vi "Hood Controller.vi"(8 "error in":errorcluster) -> ()   [LabVIEW 2019]
doc: "This VI executes continuously carrying out the current operation and responding to updates or new operations. It will often contain the timing or control code that is difficult to place directly in TeleOp. This VI generally opens all sensors and motors and isolates the rest of the robot code from knowing how the operations are carried out."
uses:
  <vilib>/Rock Robotics/WPI/Framework/Completion Status.ctl
  Hood Setpoints.ctl
  Hood Operations.ctl
  <vilib>/Rock Robotics/WPI/ThirdParty/REV Robotics/SPARK MAX/Typedef/Spark MAX Smart Motion Parameters.ctl
  <vilib>/Rock Robotics/WPI/ThirdParty/REV Robotics/SPARK MAX/Typedef/Spark MAX Control Type.ctl
  <vilib>/Rock Robotics/WPI/MotorControl/WPI_MotorControlDeviceRef.ctl
  <vilib>/Rock Robotics/WPI/MotorControl/WPI_MotorControlType.ctl
  <vilib>/Rock Robotics/SystemInterfaces/DIO/FPGA_DIOPWMChannel.ctl
  <vilib>/Rock Robotics/WPI/PWM/WPI_PWMDeadband.ctl
  <vilib>/Rock Robotics/SystemInterfaces/DIO/FPGA_DIOChannel.ctl
  <vilib>/Rock Robotics/WPI/ThirdParty/REV Robotics/SPARK MAX/Typedef/Spark MAX Motor Type.ctl
  <vilib>/Rock Robotics/WPI/ThirdParty/REV Robotics/SPARK MAX/Typedef/Spark MAX Limit Direction.ctl
panel:
  in  "Control Mode":T1=enum."Smart Motion"
  in  "Velocity PID Constants":T2={"P Gain"=2e-05, "I Gain"=0.0, "D Gain"=0.0, "F Gain"=0.0001, "I Zone"=0.0, "Min Output"=-1.0, "Max Output"=1.0} {"Max Output" min=-1.0 max=1.0 step=0.01; "Min Output" min=-1.0 max=1.0 step=0.01; "I Zone" step=0.01; "F Gain" step=0.01; "D Gain" step=0.01; "I Gain" step=0.01; "P Gain" min=0.0 step=0.01}
  in  "Smart Motion Parameters":T3={"Max Velocity"=5600.0, "Max Acceleration"=10000.0, "Minimum Velocity Output"=0.0, "Allowed Closed Loop Error"=0.001}
  in  "D Filter":dbl(slide) scale=0.0..1.0
  out "Waveform Chart":T4(graph)={"Sensor Position"=0.28571414947509766, "Sensor Velocity"=0.0, "Setpoint"=0.0}
  in  "Interactive Values":T5={"Operation"=enum."Hood Setpoint", "Setpoint"=20.0, "Duration"=0.0}
  out "Current\nCmd":string="Started at  20:35:17.047\nDefault: Reserve,  S 0.0, D 0.000000"
  in  "Buttons":cluster{"Execute Cmd":bool, "Abort Cmd":bool}
  out "Command Timing":cluster{"Start Time (ms)":u32, "Iterations":i32}={"Start Time (ms)"=6528456, "Iterations"=0}
  out "Status":T7
  # "Interactive Command: You may fill in the settings for a command\nand schedule it with the Execute button. You can observe and abort\nany command while fine tuning the code for the controller."
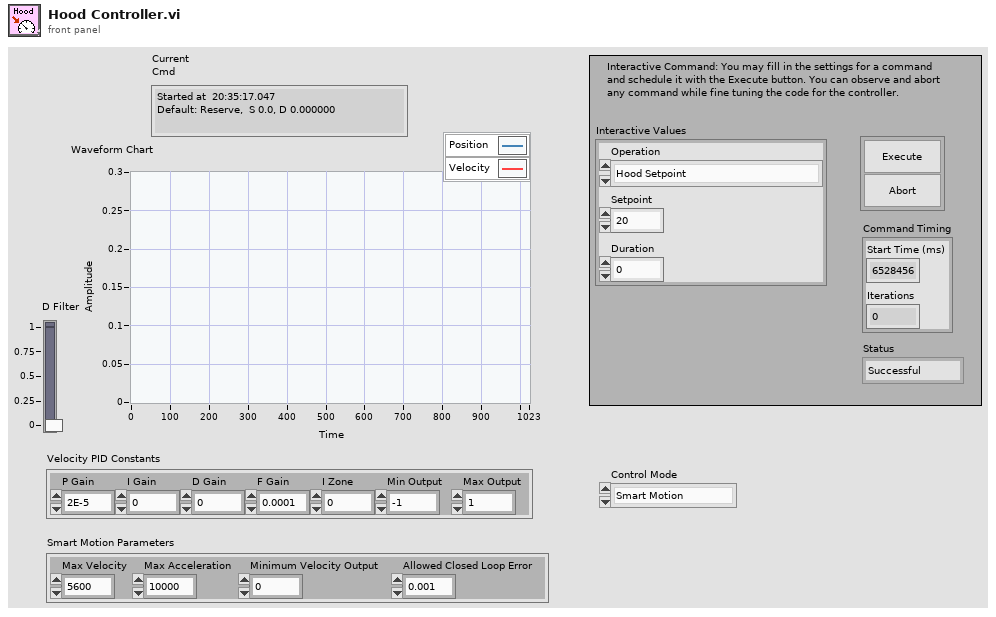
[diagram p1: front panel]
types:
  T1 = typedef "Spark MAX Control Type.ctl" = enum16{"Percent VBus", "Voltage", "Velocity", "Position", "Smart Motion", "Current", "Smart Velocity"}
  T2 = cluster{"P Gain":dbl, "I Gain":dbl, "D Gain":dbl, "F Gain":dbl, "I Zone":dbl, "Min Output":dbl, "Max Output":dbl}
  T3 = typedef "Spark MAX Smart Motion Parameters.ctl" = cluster{"Max Velocity":dbl, "Max Acceleration":dbl, "Minimum Velocity Output":dbl, "Allowed Closed Loop Error":dbl}
  T4 = cluster{"Sensor Position":dbl, "Sensor Velocity":dbl, "Setpoint":dbl}
  T5 = typedef "Hood Setpoints.ctl" = cluster{"Operation":T6, "Setpoint":dbl, "Duration":dbl}
  T6 = typedef "Hood Operations.ctl" = enum16{"Reserve", "Read Current", "Immediate", "Hood Down", "Hood Score", "Hood Setpoint"}
  T7 = typedef "Completion Status.ctl" = enum16{"Successful", "Aborted", "Incomplete"}
  T8 = typedef "Spark MAX Limit Direction.ctl" = enum16{"Forward Limit", "Reverse Limit"}
  T9 = typedef "Spark MAX Motor Type.ctl" = enum16{"Brushed", "Brushless"}
  T10 = typedef "WPI_MotorControlDeviceRef.ctl" = cluster{"DeviceStatus":errorcluster, "Type":T11, "PWM":cluster{"PWM Channel":T12, "DeadBand":T13}, "CAN":cluster{"Device Number":u8, "SetOutput VI Ref":variant, "GetOutput VI Ref":variant, "Enable VI Ref":variant, "Disable VI Ref":variant, "Data":variant}, "Invert":bool, "DIO PWM":cluster{"PWM \"Enable\" Channel":T12, "DIOChannel":T14, "PWM Rate":dbl}}
  T11 = typedef "WPI_MotorControlType.ctl" = enum16{"PWM", "CAN", "DIO PWM"}
  T12 = typedef "FPGA_DIOPWMChannel.ctl" = enum8{"PWM 0", "PWM 1", "PWM 2", "PWM 3", "PWM 4", "PWM 5", "PWM 6", "PWM 7", "PWM 8", "PWM 9", "PWM MXP 0", "PWM MXP 1", "PWM MXP 2", "PWM MXP 3", "PWM MXP 4", "PWM MXP 5", "PWM MXP 6", "PWM MXP 7", "PWM MXP 8", "PWM MXP 9", "Invalid"}
  T13 = typedef "WPI_PWMDeadband.ctl" = cluster{"Name":string, "maxPositivePwm":i32, "minPositivePwm":i32, "centerPwm":i32, "maxNegativePwm":i32, "minNegativePwm":i32, "angularRange":u16}
  T14 = typedef "FPGA_DIOChannel.ctl" = enum8{"DIO 0", "DIO 1", "DIO 2", "DIO 3", "DIO 4", "DIO 5", "DIO 6", "DIO 7", "DIO 8", "DIO 9", "DIO MXP 0", "DIO MXP 1", "DIO MXP 2", "DIO MXP 3", "DIO MXP 4", "DIO MXP 5", "DIO MXP 6", "DIO MXP 7", "DIO MXP 8", "DIO MXP 9", "DIO MXP 10", "DIO MXP 11", "DIO MXP 12", "DIO MXP 13", "DIO MXP 14", "DIO MXP 15", "SPI Port CS1", "SPI Port CS2", "SPI Port CS3", "SPI Port MISO", "SPI Port MOSI", "Invalid"}
  T15 = typedef "Command Status Info.ctl" = cluster{"Name":string, "Status":T7, "notifier out":T16}
  T16 = typedef "Completion Notifier.ctl" = refnum<notifier>
  T17 = cluster{"Current Command":T5, "Command Timing":cluster{"Start Time (ms)":u32, "Iterations":i32}, "Command Arguments":cluster{"Command Info":T15, "Description":string, "Default Command":T5, "queue out":refnum<queue>, "Subsystem Name":string}}
  T18 = cluster{"P Gain":bool, "I Gain":bool, "D Gain":bool, "F Gain":bool, "I Zone":bool, "Min Output":bool, "Max Output":bool}
  T19 = cluster{"Max Velocity":bool, "Max Acceleration":bool, "Minimum Velocity Output":bool, "Allowed Closed Loop Error":bool}
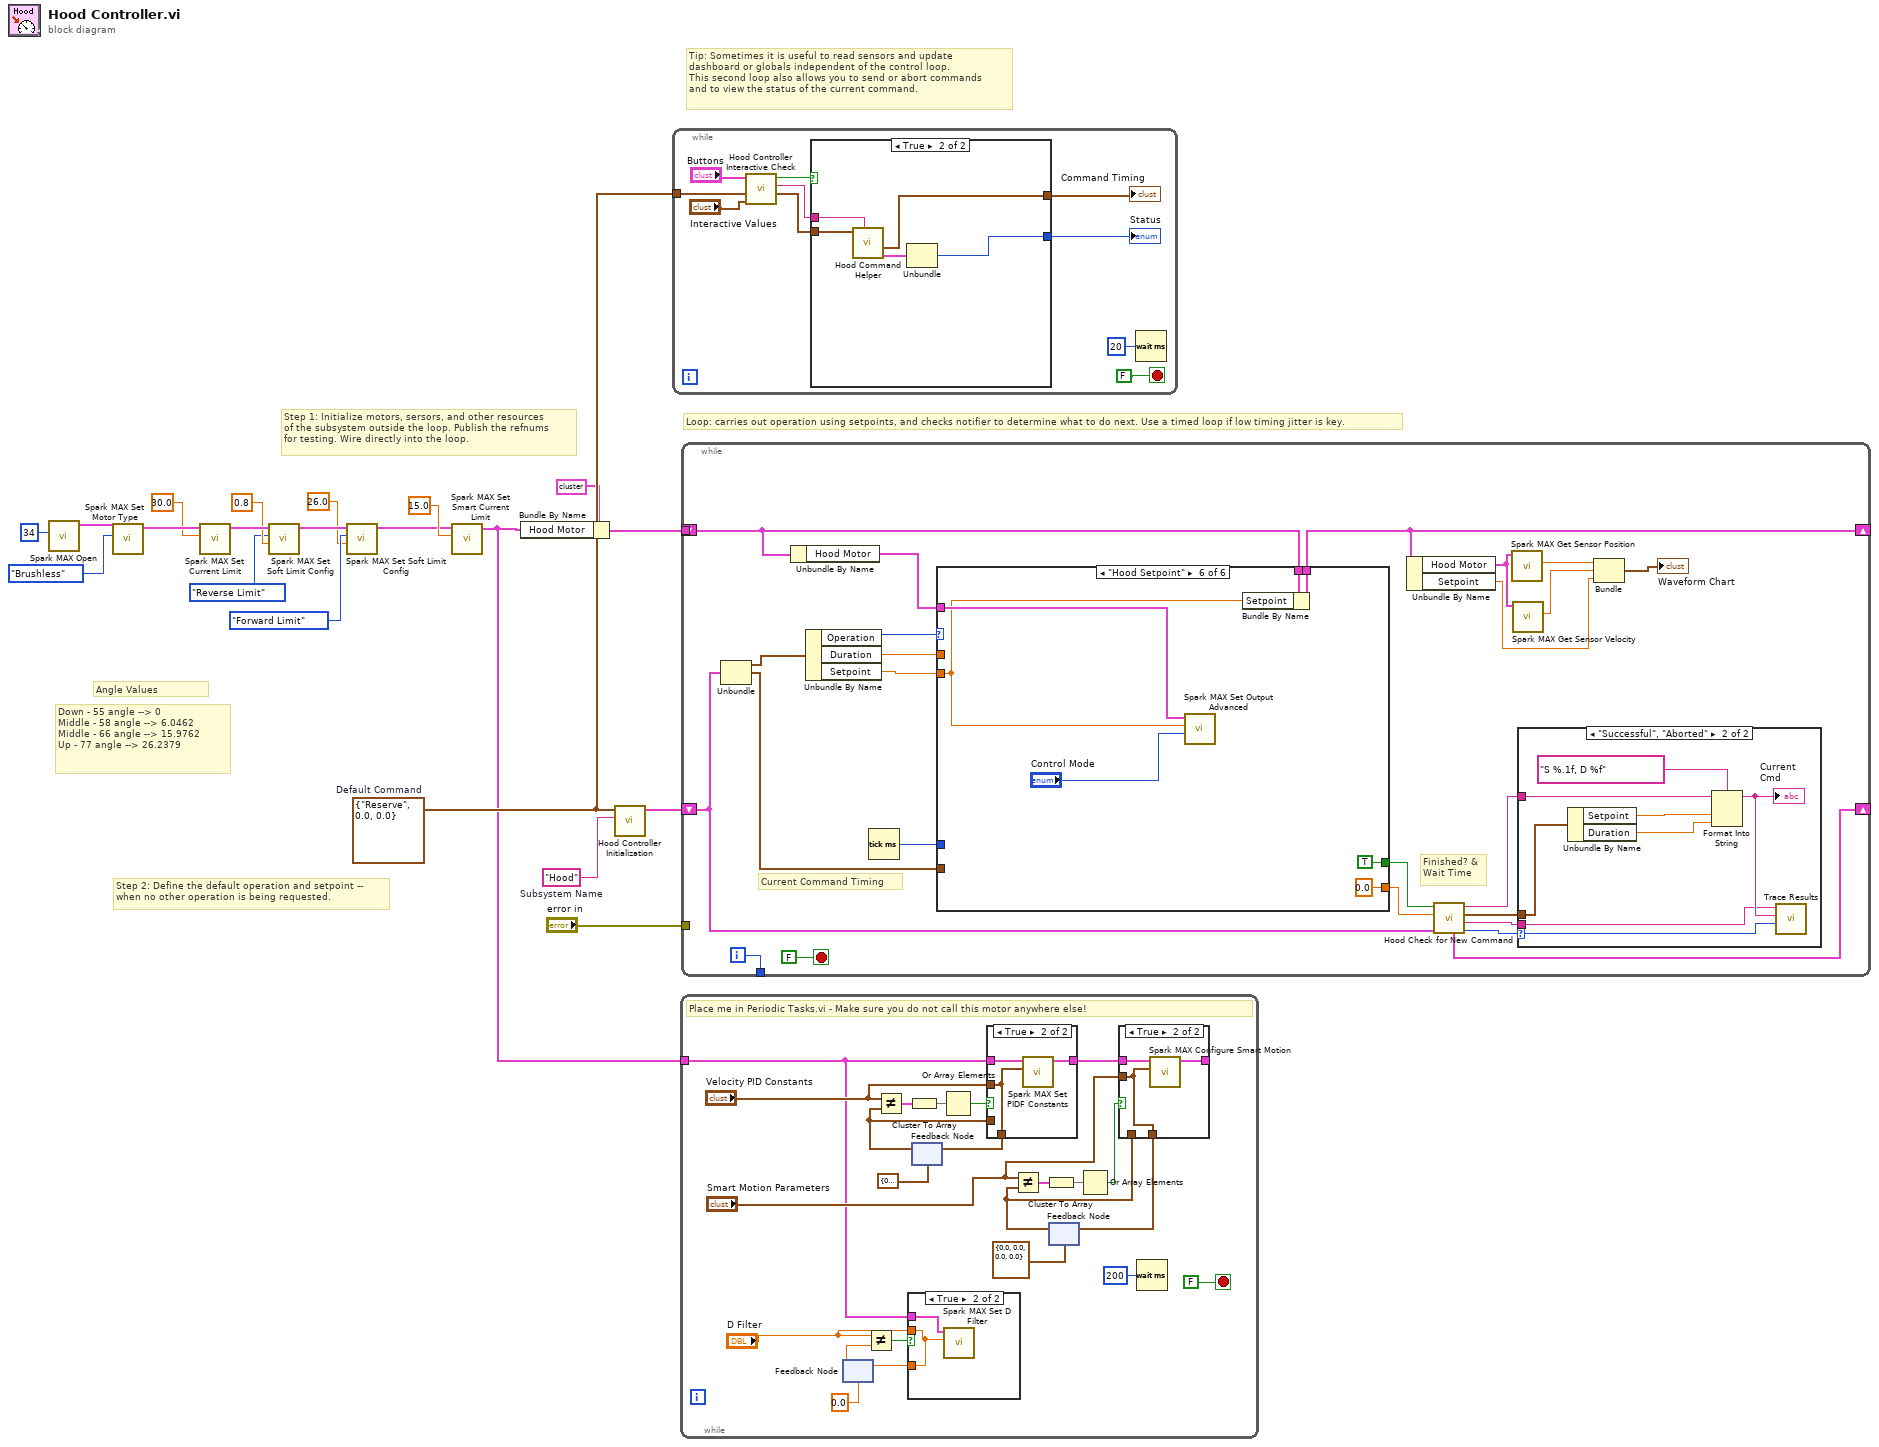
[diagram p0: block diagram]
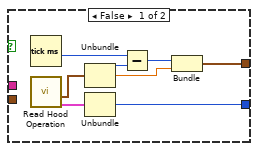
[diagram p5: hidden frame]
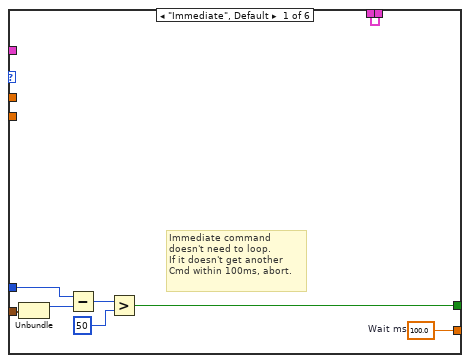
[diagram p7: hidden frame]
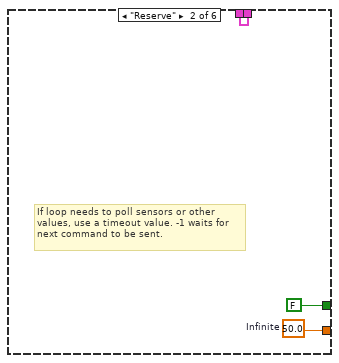
[diagram p8: hidden frame]
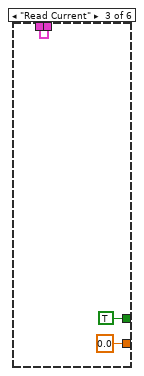
[diagram p9: hidden frame]
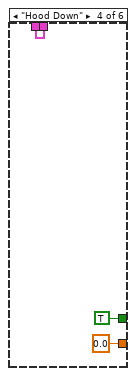
[diagram p10: hidden frame]
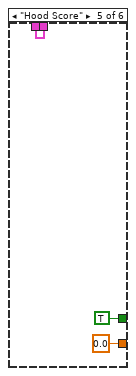
[diagram p11: hidden frame]
diagram:
  w17 = T5 {"Operation"=enum."Reserve", "Setpoint"=0.0, "Duration"=0.0}  # Default Command
  w18 = "Hood"  # Subsystem Name
  # "Angle Values"
  # "Down - 55 angle --> 0\nMiddle - 58 angle --> 6.0462\nMiddle - 66 angle --> 15.9762\nUp - 77 angle --> 26.2379"
  # "Tip: Sometimes it is useful to read sensors and update\ndashboard or globals independent of the control loop.\nThis second loop also allows you to send or abort commands\nand to view the status of the current command."
  # "Step 2: Define the default operation and setpoint --\nwhen no other operation is being requested."
  # "Step 1: Initialize motors, sersors, and other resources\nof the subsystem outside the loop. Publish the refnums\nfor testing. Wire directly into the loop."
  # "Loop: carries out operation using setpoints, and checks notifier to determine what to do next. Use a timed loop if low timing jitter is key."
  n1 = call <vilib>:"Spark MAX Open.vi"("Device Number"=u8 34) -> ("MotorControlDeviceRef"=w11:T10)  [unwired: 9 in, 1 out]
  n2 = call <vilib>:"Spark MAX Set Motor Type.vi"("Motor Type"=Spark_MAX_Motor_Type."Brushless", "MotorControlDevRef"=w11) -> ("MotorControlDeviceRef"=w15:T10)  [unwired: 8 in, 1 out]
  n3 = call <vilib>:"Spark MAX Set Current Limit.vi"("Current Limit A (100)"=sgl 30.0, "MotorControlDeviceRef in"=w15) -> ("MotorControlDeviceRef out"=w8:T10)  [unwired: 8 in, 1 out]
  n4 = call <vilib>:"Spark MAX Set Soft Limit Config.vi"("Soft Limit (0)"=0.8, "Soft Limit Switch"=Spark_MAX_Limit_Direction."Reverse Limit", "MotorControlDeviceRef in"=w8) -> ("MotorControlDeviceRef out"=w7:T10)  [unwired: 7 in, 1 out]
  n5 = call <vilib>:"Spark MAX Set Soft Limit Config.vi"("Soft Limit (0)"=26.0, "Soft Limit Switch"=Spark_MAX_Limit_Direction."Forward Limit", "MotorControlDeviceRef in"=w7) -> ("MotorControlDeviceRef out"=w4:T10)  [unwired: 7 in, 1 out]
  n6 = call <vilib>:"Spark MAX Set Smart Current Limit.vi"("Primay Current Limit (80A)"=15.0, "MotorControlDeviceRef in"=w4) -> ("MotorControlDeviceRef out"=w1:T10)  [unwired: 8 in, 1 out]
  n7 = Bundle By Name(cluster=cluster{"Hood Motor":T10, "Setpoint":dbl} {"Hood Motor"={"DeviceStatus"={"status"=FALSE, "code"=0, "source"=""}, "Type"=enum."PWM", "PWM"={"PWM Channel"=enum."Invalid", "DeadBand"={"Name"="", "maxPositivePwm"=0, "minPositivePwm"=0, "centerPwm"=0, "maxNegativePwm"=0, "minNegativePwm"=0, "angularRange"=0}}, "CAN"={"Device Number"=0, "SetOutput VI Ref"=variant(refnum<vi> refnum), "GetOutput VI Ref"=variant(refnum<vi> refnum), "Enable VI Ref"=variant(refnum<vi> refnum), "Disable VI Ref"=variant(refnum<vi> refnum), "Data"=variant}, "Invert"=FALSE, "DIO PWM"={"PWM \"Enable\" Channel"=enum."Invalid", "DIOChannel"=enum."Invalid", "PWM Rate"=0.0}}, "Setpoint"=0.0} ("input cluster"), "Hood Motor"=w1) -> (w10:cluster{"Hood Motor":T10, "Setpoint":dbl})
  n8 = call "Hood Controller Initialization.vi"("Subsystem Name"=w18, "Default Command"=w17) -> ("Current Command"=w19:T17)  [unwired: 9 in]
  n9 = while {
    tunnel: w17 -> [w27]
    stop <- FALSE stop-if-true
    n10 = call "Hood Controller Interactive Check.vi"("Interactive Command in"="Interactive Values", "Default Command"=w27, "Buttons"="Buttons") -> ("Interactive Command out"=w24:T5, "Trace String"=w25:string, "Schedule"=w26:bool)  [unwired: 6 in]
    n11 = case shown="True" w26 {
      tunnel: [w38 w43] -> w23
      tunnel: w24 -> [_ w41]
      tunnel: [w34 w39] -> w22
      tunnel: w25 -> [_ w42]
      frame False {
        n12 = Tick Count (ms)() -> (millisecond timer value=w33:u32)
        n13 = call "Read Hood Operation.vi"() -> ("Command Info"=w31:T15, "SubSystem Data"=w32:T5)  [unwired: 9 in, 1 out]
        n14 = Unbundle(w32) -> ("Operation"=w37:T6, "Setpoint"=w35:dbl)  [unwired: 1 out]
        n15 = Unbundle(w31) -> ("Status"=w38:T7)  [unwired: 2 out]
        n16 = Subtract(x=w33, y=w37) -> (x-y=w36:u32)
        n17 = Bundle(w36, "Setpoint"=w35) -> (w34:cluster{u32, "Setpoint":dbl})  [unwired: 1 in]
      }
      frame True {
        n18 = call "Hood Command Helper.vi"("Description"=w42, "SubSystem Data"=w41) -> ("Command Info Out"=w40:T15, "Command Timing"=w39:cluster{"Start Time (ms)":u32, "Iterations":i32})  [unwired: 7 in, 1 out]
        n19 = Unbundle(w40) -> ("Status"=w43:T7)  [unwired: 2 out]
      }
    }
    "Status" <- w23
    "Command Timing" <- w22
    n20 = Wait (ms)(milliseconds to wait=u32 20) -> ()  [unwired: 1 out]
  }
  n21 = while {
    tunnel: w1 -> [w46]
    stop <- FALSE stop-if-true
    # "Place me in Periodic Tasks.vi - Make sure you do not call this motor anywhere else!"
    n22 = feedback #1(0.0) -> (w47:dbl)
    n23 = Not Equal?(x="D Filter", y=w47) -> (x != y?=w48:bool)
    n24 = case shown="True" w48 {
      tunnel: w46 -> [_ w69]
      tunnel: "D Filter" -> [w67 w68]
      tunnel: [w67 w68] -> w44
      frame False {
      }
      frame True {
        n25 = call <vilib>:"Spark MAX Set D Filter.vi"("Derivative Filter (0)"=w68, "MotorControlDeviceRef in"=w69) -> ()  [unwired: 8 in, 2 out]
      }
    }
    n26 = feedback-in #1(w44) -> ()
    n27 = feedback #2(T2 {"P Gain"=0.0, "I Gain"=0.0, "D Gain"=0.0, "F Gain"=0.0, "I Zone"=0.0, "Min Output"=0.0, "Max Output"=0.0} ("PID Constants")) -> (w66:T2)
    n28 = Not Equal?(x="Velocity PID Constants", y=w66) -> (x != y?=w60:T18)
    n29 = Cluster To Array(cluster=w60) -> (array=w61:bool[])
    n30 = Or Array Elements(Boolean array=w61) -> (logical OR=w63:bool)
    n31 = case shown="True" w63 {
      tunnel: w46 -> [w75 w79]
      tunnel: "Velocity PID Constants" -> [_ w77]
      tunnel: [w76 w77] -> w65
      tunnel: w66 -> [w76 _]
      tunnel: [w75 w78] -> w57
      frame False {
      }
      frame True {
        n32 = call <vilib>:"Spark MAX Set PIDF Constants.vi"("PID Constants"=w77, "MotorControlDeviceRef"=w79) -> ("MotorControlDeviceRef"=w78:T10)  [unwired: 8 in, 1 out]
      }
    }
    n33 = feedback-in #2(w65) -> ()
    n34 = feedback #3(T3 {"Max Velocity"=0.0, "Max Acceleration"=0.0, "Minimum Velocity Output"=0.0, "Allowed Closed Loop Error"=0.0} ("Smart Motion Parameters")) -> (w50:T3)
    n35 = Not Equal?(x="Smart Motion Parameters", y=w50) -> (x != y?=w55:T19)
    n36 = Cluster To Array(cluster=w55) -> (array=w56:bool[])
    n37 = Or Array Elements(Boolean array=w56) -> (logical OR=w54:bool)
    n38 = case shown="True" w54 {
      tunnel: w57 -> [w71 w74]
      tunnel: "Smart Motion Parameters" -> [_ w72]
      tunnel: [w71 w73] -> _
      tunnel: [w70 w72] -> w51
      tunnel: w50 -> [w70 _]
      frame False {
      }
      frame True {
        n39 = call <vilib>:"Spark MAX Configure Smart Motion.vi"("Smart Motion Parameters"=w72, "MotorControlDeviceRef"=w74) -> ("MotorControlDeviceRef"=w73:T10)  [unwired: 8 in, 1 out]
      }
    }
    n40 = feedback-in #3(w51) -> ()
    n41 = Wait (ms)(milliseconds to wait=u32 200) -> ()  [unwired: 1 out]
  }
  n42 = while {
    shift-right: [w95] -> _
    shift-left: w19 -> [w88]
    tunnel: [w102] -> _
    tunnel: "error in" -> [_]
    tunnel: w10 -> [w83]
    shift-right: [w82] -> _
    shift-left: _ -> [_]
    i -> [w102]
    stop <- FALSE stop-if-true
    # "Current Command Timing"
    # "Finished? &\nWait Time"
    n43 = Unbundle(w88) -> ("Current Command"=w101:T5, "Command Timing"=w97:cluster{"Start Time (ms)":u32, "Iterations":i32})  [unwired: 1 out]
    n44 = Unbundle By Name(w83) -> ("Hood Motor"=w85:T10)
    n45 = Unbundle By Name(w101) -> ("Operation"=w100:T6, "Duration"=w99:dbl, "Setpoint"=w96:dbl)
    n46 = Tick Count (ms)() -> (millisecond timer value=w98:u32)
    n47 = case shown="\"Hood Setpoint\"" w100 {
      tunnel: [w119 w122 0.0 ("Infinite") 0.0 ("Infinite") 0.0 ("Infinite") 0.0 ("Infinite")] -> w93
      tunnel: [w113 FALSE ("ignore previous (F)") TRUE ("ignore previous (F)") TRUE ("ignore previous (F)") TRUE ("ignore previous (F)") TRUE ("ignore previous (F)")] -> w94
      tunnel: w97 -> [w115 _ _ _ _ _]
      tunnel: w99 -> [_ _ _ _ _ _]
      tunnel: w98 -> [w114 _ _ _ _ _]
      tunnel: w96 -> [_ _ _ _ _ w132]
      tunnel: w85 -> [_ _ _ _ _ w137]
      tunnel: w83 -> [w112 w120 w123 w126 w129 w134]
      tunnel: [w112 w120 w123 w126 w129 w133] -> w82
      frame "Immediate", Default {
        w119 = 100.0  # Wait ms
        # "Immediate command\ndoesn't need to loop.\nIf it doesn't get another\nCmd within 100ms, abort."
        n48 = Unbundle(w115) -> ("Start Time (ms)"=w118:u32)  [unwired: 1 out]
        n49 = Subtract(x=w114, y=w118) -> (x-y=w117:u32)
        n50 = Greater?(x=w117, y=u8 50 ("Left Motor")) -> (0:w113:bool)
      }
      frame "Reserve" {
        w122 = 50.0  # Infinite
        # "If loop needs to poll sensors or other\nvalues, use a timeout value. -1 waits for\nnext command to be sent."
      }
      frame "Read Current" {
      }
      frame "Hood Down" {
      }
      frame "Hood Score" {
      }
      frame "Hood Setpoint" {
        n51 = call <vilib>:"Spark MAX Set Output Advanced.vi"("Control Mode"="Control Mode", "Setpoint"=w132, "MotorControlDevRef"=w137) -> ()  [unwired: 7 in, 2 out]
        n52 = Bundle By Name(cluster=w134, "Setpoint"=w132) -> (w133:cluster{"Hood Motor":T10, "Setpoint":dbl})
      }
    }
    n53 = Unbundle By Name(w82) -> ("Hood Motor"=w81:T10, "Setpoint"=w80:dbl)
    n54 = call "Hood Check for New Command.vi"("Current Command"=w88, "Wait time (ms)"=w93, "Finished?"=w94) -> ("Completion"=w89:T7, "Subsystem Name"=w90:string, "Current Command"=w91:T5, "Initial Trace String"=w92:string, "NextCommand"=w95:T17)  [unwired: 4 in]
    n55 = call <vilib>:"Spark MAX Get Sensor Position.vi"("MotorControlDevRef in"=w81) -> ("Sensor Position"=w87:dbl)  [unwired: 7 in, 3 out]
    n56 = call <vilib>:"Spark MAX Get Sensor Velocity.vi"("MotorControlDevRef in"=w81) -> ("Sensor Velocity"=w84:dbl)  [unwired: 7 in, 3 out]
    n57 = case shown="\"Successful\", \"Aborted\"" w89 {
      selector: w89 -> [_ w111]
      tunnel: w92 -> [_ w107]
      tunnel: w91 -> [_ w108]
      tunnel: w90 -> [_ w104]
      frame "Incomplete", Default {
        # "Continuing current command"
      }
      frame "Successful", "Aborted" {
        # "Report and setup for next command"
        n58 = Unbundle By Name(w108) -> ("Setpoint"=w110:dbl, "Duration"=w105:dbl)
        n59 = Format Into String(format string="S %.1f, D %f", initial string=w107, w110, w105) -> (resulting string=w106:string)  [unwired: 1 in, 1 out]
        "Current\nCmd" <- w106
        n60 = call <vilib>:"Trace Results.vi"("Status of previous command"=w111, "Description"=w106, "Subsystem"=w104) -> ()  [unwired: 9 in]
      }
    }
    n61 = Bundle("Sensor Position"=w87, "Sensor Velocity"=w84, "Setpoint"=w80) -> (→"Waveform Chart":T4)  [unwired: 1 in]
  }
